vi "VI, Grow Panel Width.vi"(5 "margin (20)":i16=20, 6 "error in":errorcluster, 9 "VI ref":refnum<vi>) -> (0 "error out":errorcluster, 3 "VI ref dup":refnum<vi>)   [LabVIEW 2010]
doc: "This function increases a panels width to display all controls on a panel."
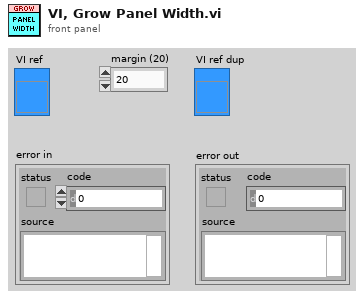
[diagram p1: front panel]
types:
  T1 = typedef "LVRectTypeDef.ctl" = cluster{"left":i16, "top":i16, "right":i16, "bottom":i16}
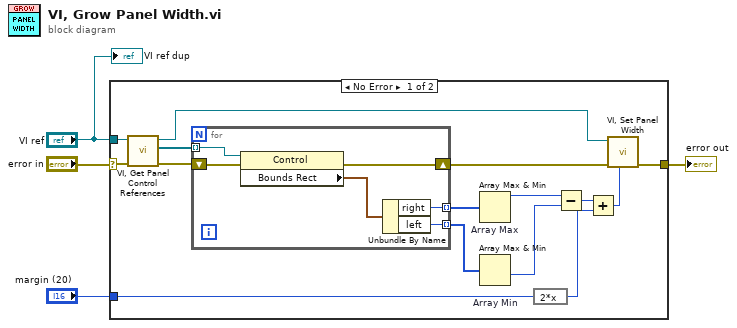
[diagram p0: block diagram]
diagram:
  n1 = case shown="No Error" "error in" {
    selector: "error in" -> [w9 w26]
    tunnel: "VI ref" -> [w8 _]
    tunnel: [w14 w26] -> w2
    tunnel: "margin (20)" -> [w10 _]
    frame No Error {
      n2 = call "VI, Get Panel Control References.vi"("error in"=w9, "VI ref"=w8) -> ("error out"=w7:errorcluster, "Ctl refnum array"=w5:refnum<vi>[], "VI ref dup"=w6:refnum<vi>)  [unwired: 5 in]
      n3 = for {
        tunnel: [w24] -> w19 mode=indexing
        tunnel: [w23] -> w18 mode=indexing
        shift-right: [w22] -> w15
        shift-left: w7 -> [w21]
        tunnel: w5 -> [w20] mode=indexing
        n4 = property class="Control"(reference=w20, error in=w21) -> (error out=w22:errorcluster, "Bounds Rect"=w25:T1)  [unwired: 1 out]
        n5 = Unbundle By Name(w25) -> ("right"=w24:i16, "left"=w23:i16)
      }
      n6 = Array Max & Min "Array Max"(array=w19) -> (max value=w17:i16)  [unwired: 3 out]
      n7 = Array Max & Min "Array Min"(array=w18) -> (min value=w16:i16)  [unwired: 3 out]
      n8 = expression code="2*x"(w10) -> (w11:i16)
      n9 = Subtract(x=w17, y=w16) -> (x-y=w13:i16)
      n10 = Add(x=w13, y=w11) -> (x+y=w12:i16)
      n11 = call "VI, Set Panel Width.vi"("width"=w12, "error in"=w15, "VI ref"=w6) -> ("error out"=w14:errorcluster)  [unwired: 5 in, 1 out]
    }
    frame Error {
    }
  }
  "error out" <- w2
  "VI ref dup" <- "VI ref"
